vi "ControlSystem_Creator.vi"(12 "Desired Poles":cdb[](array[numeric])=[-5.0+0.0i, -5.0+0.0i, -20.0+0.0i, -15.0+0.0i] format="%#.2g", 13 "Stop Button":bool) -> (3 "Sampling Time Required":dbl=0.1 format="%.2f", 4 "System Poles":cdb[](array[numeric])=[1.2142841528821395+0.0i, 0.8147971273698099+0.0i, 0.9518587677710494+0.0i, 1.0+0.0i] format="%#.2g", 6 "Feedback Gain (K)":dbl[](array[numeric])=[-63312112.22140336, 6720868.965421855, 193328496.30508494, -20246021.6652911], 8 "Controllability Matrix":dbl[][](array[numeric])=[[0.0029424877498334255, 0.008616646869548867, 0.014016016852462686, 0.019193532183387766], [0.05829906495647488, 0.05527735475623796, 0.052797981566245, 0.05083784073300338], [0.000983525405599516, 0.0029123179012991098, 0.004844756877997715, 0.006861898357198368], [0.019540617662783182, 0.019171356382024756, 0.019611979984952656, 0.02086921364939449]] format="%.2f", 10 "Discrete State-Space Model":T5={"properties"={"Model name"="System Model", "Input names"=["u0"], "Output names"=["y0"], "Input Delays"=[0.0], "Output Delays"=[0.0], "Sampling Time"=0.1, "Notes"=""}, "A"=[[1.0, 0.09705751225016658, 0.009648384228931255, 0.00032278803187467067], [0.0, 0.9417009350435251, 0.19169345927190307, 0.009648384228931255], [0.0, -0.0009835254055995163, 1.019619556489737, 0.10065366453071445], [0.0, -0.019540617662783182, 0.39303530277273724, 1.019619556489737]], "B"=[[0.0029424877498334255], [0.05829906495647488], [0.000983525405599516], [0.019540617662783182]], "C"=[[0.0, 0.0, 1.0, 0.0]], "D"=[[0.0]], "StateNames"=["x0", "x1", "x2", "x3"], "Transport Delay"=[[0.0]]} {"Transport Delay" format="%.2f"; "D" format="%#.2g"; "C" format="%#.2g"; "B" format="%#.2g"; "A" format="%#.2g"; "properties"."Sampling Time" format="%#.6p"; "properties"."Output Delays" format="%.4f"; "properties"."Input Delays" format="%.4f"}, 14 "Calculated Poles":cdb[](array[numeric])=[-20.00002973836509+0.0i, -14.99996105048431+0.0i, -5.004299732705596+0.0i, -4.995709482028461+0.0i] format="%#.2g", 15 "Discrete Model Out":picture)   [LabVIEW 2012]
uses:
  <vilib>/addons/Control Design/_Model Construction/Model Typedefs.llb/CD State Space Model (MIMO).ctl
  <vilib>/addons/Control Design/_Model Construction/Model Typedefs.llb/CD General Elements.ctl
  <vilib>/addons/Control Design/_Model Construction/Model Typedefs.llb/CD Zero-Pole-Gain Model (MIMO).ctl
  <vilib>/addons/Control Design/_Model Construction/Model Typedefs.llb/CD Zero-Pole-Gain Model (SISO).ctl
  <vilib>/addons/Control Design/_Model Construction/Data Typedefs.llb/CD Model Type.ctl
  <vilib>/addons/Control Design/_Model Construction/Model Creation.llb/Model Creation SubVI/cd_Create State Space Model.vi
  <vilib>/addons/Control Design/_Time Response Analysis/Time Response.llb/Time Response subVI/cd_Step Response (State-Space).vi
  <vilib>/addons/Control Design/_Utility/Model Viewer.llb/Model Viewer SubVI/cd_Draw State-Space Equation (SS).vi
  <vilib>/addons/Control Design/_Dynamic Analysis/Dynamic Analysis.llb/Dynamic Analysis subVI/cd_Pole-Zero Map (State-Space).vi
  <vilib>/addons/Control Design/_Model Conversions/Model Type.llb/Model Conversion SubVI/cd_Convert State-Space to Zero-Pole-Gain Model.vi
  <vilib>/addons/Control Design/_Model Construction/Model Information.llb/Model Information SubVIs/cd_Verify If Discrete (State-Space).vi
  <vilib>/addons/Control Design/_Model Construction/Model Information.llb/Model Information SubVIs/cd_Check State Space Model.vi
  <vilib>/addons/Control Design/_Model Construction/Model Information.llb/Model Information SubVIs/cd_Verify Model Type (SS).vi
  <vilib>/addons/Control Design/_Dynamic Analysis/Dynamic Analysis.llb/Dynamic Analysis subVI/cd_Poles (State-Space).vi
  <vilib>/addons/Control Design/_Model Conversions/Continuous and Discrete.llb/Continuous and Discrete SubVI/cd_Convert Continuous to Discrete (SS).vi
  <vilib>/addons/Control Design/_State Feedback Control/NI_CD_State Feedback Control.lvlib
  <vilib>/addons/Control Design/_Dynamic Analysis/NI_CD_Dynamic Analysis.lvlib
  <vilib>/addons/Control Design/_Model Conversions/NI_CD_Continuous and Discrete.lvlib
  <vilib>/addons/Control Design/_State-Space Analysis/NI_CD_State-Space Analysis.lvlib
  <vilib>/addons/Control Design/_Model Construction/NI_LinSys_Model Information.lvlib
  <vilib>/addons/Control Design/_Model Conversions/NI_CD_Model Type.lvlib
  <vilib>/addons/Control Design/_Model Construction/NI_LinSys_Model Creation.lvlib
  <vilib>/addons/Control Design/_Utility/NI_CD_Model Viewer.lvlib
  <vilib>/addons/Control Design/_Time Response Analysis/NI_CD_Time Response.lvlib
  <vilib>/addons/Control Design/_Model Construction/NI_LinSys_Model Typedefs.lvlib
  <vilib>/addons/Control Design/_Model Construction/NI_LinSys_Data Typedefs.lvlib
panel:
  in  "x":bool
  in  "Sampling Time (s)":dbl=0.1
  in  "Discrete Mode":bool=TRUE
  out "Number of States":i32=4
  out "Number of Inputs":i32=1
  out "Number of Outputs":i32=1
  out "Type of Model":T1=1 items=["Empty", "SISO", "SIMO", "MISO", "MIMO", "Undetermined"]
  out "Discrete?":bool=TRUE
  out "Static Gain Case?":bool
  out "Zero-Pole-Gain Model":T2={"properties"={"Model name"="System Model", "Input names"=["u0"], "Output names"=["y0"], "Input Delays"=[0.0], "Output Delays"=[0.0], "Sampling Time"=0.1, "Notes"=""}, "zero-pole-gain(s)"=[[{"Gain"=0.000983525405599206, "Zeros"=[0.999999999999886+0.0i, -0.9801607885382041+0.0i], "Poles"=[0.8147971273698099+0.0i, 0.9518587677710494+0.0i, 1.2142841528821395+0.0i], "delay"=0.0}]]} {"zero-pole-gain(s)"."delay" format="%.4f"; "zero-pole-gain(s)"."Poles" format="%#.8g"; "zero-pole-gain(s)"."Zeros" format="%#.8g"; "zero-pole-gain(s)"."Gain" format="%#.8g"; "properties"."Sampling Time" format="%#.6p"; "properties"."Output Delays" format="%.4f"; "properties"."Input Delays" format="%.4f"}
  out "Pole-Zero Map":cluster{dbl[], dbl[]}[](graph)=[{[1.2142841528821395, 0.8147971273698099, 0.9518587677710494, 1.0], [0.0, 0.0, 0.0, 0.0]}, {[1.0, 1.0, -0.980160788537376], [0.0, 0.0, 0.0]}]
  out "Step Response Graph":cluster{"time":dbl[], dbl[]}[](graph)
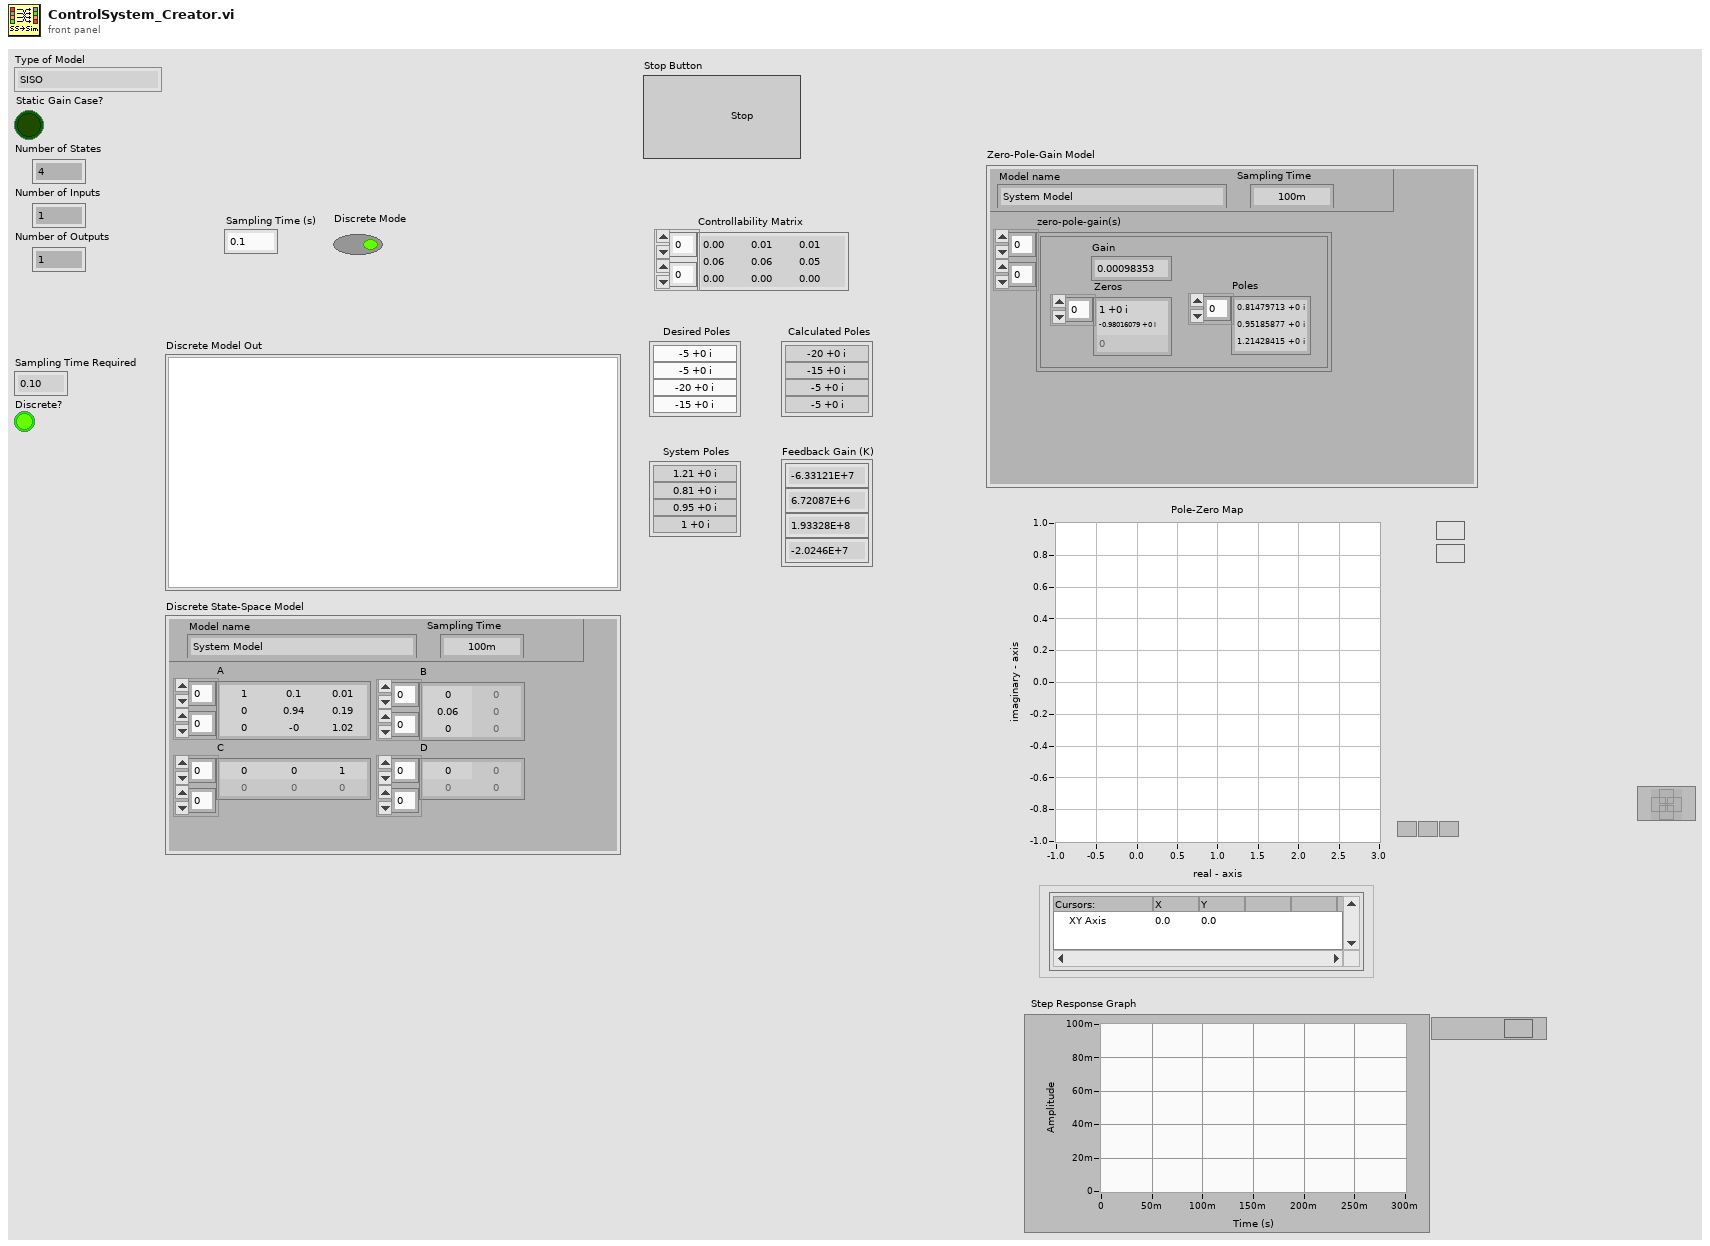
[diagram p1: front panel]
types:
  T1 = typedef "NI_LinSys_Data Typedefs.lvlib/CD Model Type.ctl" = u16
  T2 = typedef "NI_LinSys_Model Typedefs.lvlib/CD Zero-Pole-Gain Model (MIMO).ctl" = cluster{"properties":T3, "zero-pole-gain(s)":T4[][]}
  T3 = typedef "NI_LinSys_Model Typedefs.lvlib/CD General Elements.ctl" = cluster{"Model name":string, "Input names":string[], "Output names":string[], "Input Delays":dbl[], "Output Delays":dbl[], "Sampling Time":dbl, "Notes":string}
  T4 = typedef "NI_LinSys_Model Typedefs.lvlib/CD Zero-Pole-Gain Model (SISO).ctl" = cluster{"Gain":dbl, "Zeros":cdb[], "Poles":cdb[], "delay":dbl}
  T5 = typedef "NI_LinSys_Model Typedefs.lvlib/CD State Space Model (MIMO).ctl" = cluster{"properties":T3, "A":dbl[][], "B":dbl[][], "C":dbl[][], "D":dbl[][], "StateNames":string[], "Transport Delay":dbl[][]}
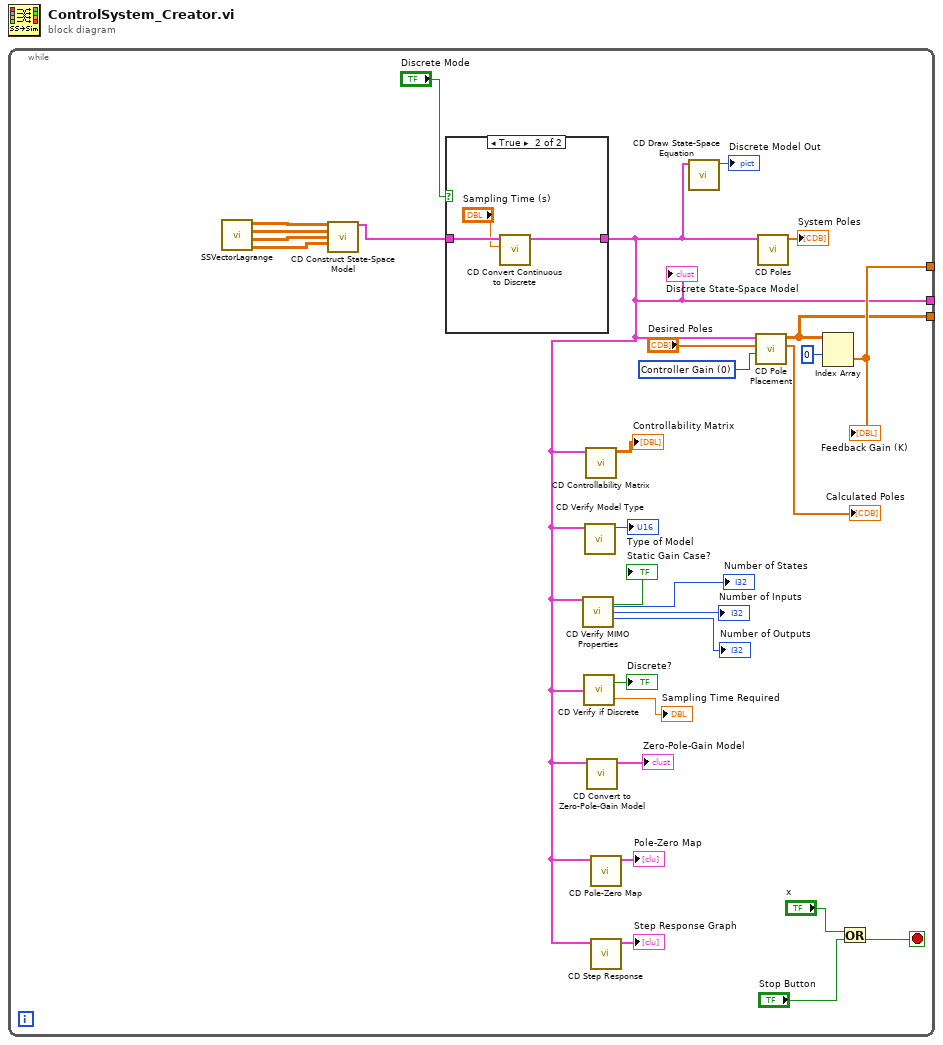
[diagram p0: block diagram]
diagram:
  n1 = while {
    tunnel: [w24] -> _
    tunnel: [w11] -> _
    tunnel: [w9] -> _
    stop <- w6 stop-if-true
    w29 = u16 0 items=["Controller Gain", "Observer Gain (Predictive)", "Observer Gain (Current)"] ("Gain Type")
    n2 = call "SSVectorLagrange.vi"() -> ("D"=w1:dbl[][], "C"=w2:dbl[][], "B"=w3:dbl[][], "A"=w4:dbl[][])  [unwired: 5 in]
    n3 = call-poly <vilib>:"CD Construct State-Space Model.vi"("A"=w4, "B"=w3, "C"=w2, "D"=w1) -> ("State-Space Model"=w23:T5)  [unwired: 10 in, 1 out]
    n4 = case shown="True" "Discrete Mode" {
      tunnel: w23 -> [w30 w33]
      tunnel: [w30 w31] -> w9
      frame False {
      }
      frame True {
        n5 = call-poly <vilib>:"CD Convert Continuous to Discrete.vi"("Sampling Time (s)"="Sampling Time (s)", "Continuous State-Space Model"=w33) -> ("Discrete State-Space Model"=w31:T5)  [unwired: 7 in, 2 out]
      }
    }
    "Discrete State-Space Model" <- w9
    n6 = call-poly <vilib>:"CD Verify MIMO Properties.vi"("State-Space Model In"=w9) -> ("Static Gain Case?"=→"Static Gain Case?":bool, "Number of States"=→"Number of States":i32, "Number of Inputs"=→"Number of Inputs":i32, "Number of Outputs"=→"Number of Outputs":i32)  [unwired: 9 in, 2 out]
    n7 = call-poly <vilib>:"CD Verify if Discrete.vi"("State-Space Model"=w9) -> ("Discrete?"=→"Discrete?":bool, "Sampling Time"=→"Sampling Time Required":dbl)
    n8 = call-poly <vilib>:"CD Verify Model Type.vi"("State-Space Model"=w9) -> ("Type of Model"=→"Type of Model":T1)  [unwired: 9 in, 1 out]
    n9 = call <vilib>:"CD Controllability Matrix.vi"("State-Space Model"=w9) -> ("Controllability Matrix"=→"Controllability Matrix":dbl[][])  [unwired: 7 in, 3 out]
    n10 = call-poly <vilib>:"CD Convert to Zero-Pole-Gain Model.vi"("State-Space Model"=w9) -> ("Zero-Pole-Gain Model"=→"Zero-Pole-Gain Model":T2)  [unwired: 9 in, 1 out]
    n11 = call-poly <vilib>:"CD Pole-Zero Map.vi"("State-Space Model"=w9) -> ("Pole-Zero Map"=→"Pole-Zero Map":cluster{dbl[], dbl[]}[])  [unwired: 7 in, 3 out]
    n12 = call-poly <vilib>:"CD Step Response.vi"("State-Space Model"=w9) -> ("Step Response Graph"=→"Step Response Graph":cluster{"time":dbl[], dbl[]}[])  [unwired: 7 in, 3 out]
    n13 = call-poly <vilib>:"CD Draw State-Space Equation.vi"("State-Space Model"=w9) -> ("Equation"=→"Discrete Model Out":picture)  [unwired: 8 in, 2 out]
    n14 = call <vilib>:"CD Pole Placement.vi"("Gain Type"=w29, "Poles"="Desired Poles", "State-Space Model"=w9) -> ("Actual Poles"=→"Calculated Poles":cdb[], "Gain"=w11:dbl[][])  [unwired: 6 in, 1 out]
    n15 = call-poly <vilib>:"CD Poles.vi"("State-Space Model"=w9) -> ("Poles"=→"System Poles":cdb[])  [unwired: 9 in, 1 out]
    n16 = Index Array(array=w11, index (row)=0) -> (element=w24:dbl[])  [unwired: 1 in]
    "Feedback Gain (K)" <- w24
    n17 = Or(x="x", y="Stop Button") -> (x .or. y?=w6:bool)
  }
